vi "Network Steam Read Messages.vi"(8 "error in (no error)":errorcluster, 11 "Model in":refnum<class "Model.lvclass">) -> (0 "error out":errorcluster, 1 "Messages":T1[](array[typedef]), 2 "StillConnected?":bool, 3 "Model out":refnum<class "Model.lvclass">, 4 "Timed Out?":bool)   [LabVIEW 2021, in "Model.lvlib" / "Model.lvclass"]
uses:
  Model.lvclass
  Model.lvclass/Model.ctl
  <userlib>/John_Lib/Network_Streams_Connection/NetworkConnection.lvclass
  4d02eaad-354f-40a9-9b46-312da8ef89df.vi
  <userlib>/John_Lib/Network_Streams_Connection/NetworkCommand--Cluster.ctl
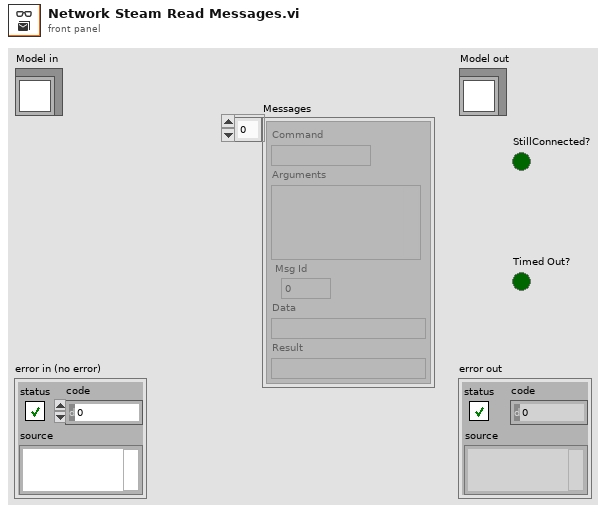
[diagram p1: front panel]
types:
  T1 = typedef "JKI_Network_Streams.lvlib/NetworkConnection.lvclass/NetworkCommand--Cluster.ctl" = cluster{"Command":string, "Arguments":variant, " Msg Id":i32, "Data":string, "Result":string}
  T2 = typedef "Model.lvlib/Model.lvclass/DVR.ctl" = cluster{"JKI_Network_Streams":refnum<class "NetworkConnection.lvclass">}
  T3 = typedef "AMC_FW.lvlib/Queue.ctl" = cluster{"Q":T4, "Name":string}
  T4 = typedef "AMC_FW.lvlib/Message Queue.ctl" = refnum<queue>
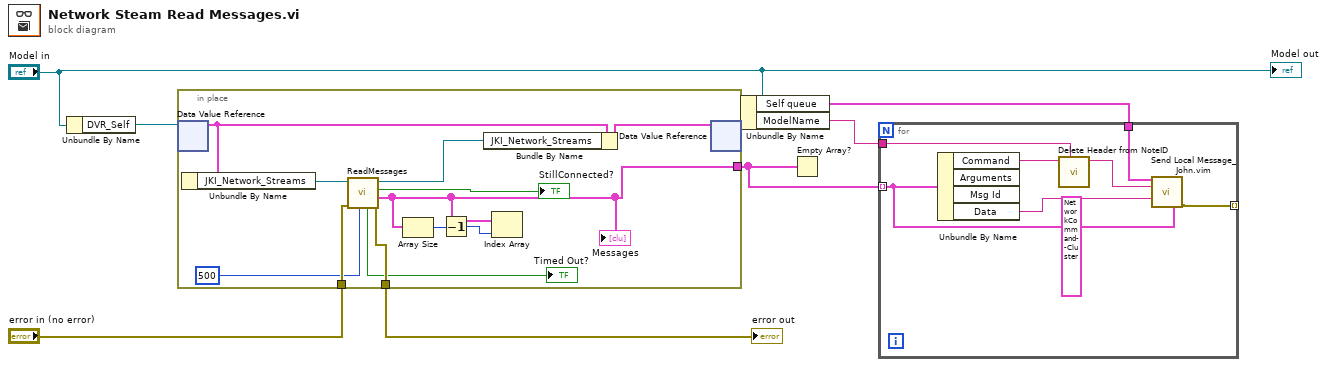
[diagram p0: block diagram]
diagram:
  n1 = Unbundle By Name("Model in") -> ("DVR_Self"=w7:refnum<data-value>)
  n2 = in-place {
    in-place-border: "error in (no error)" -> [w15]
    in-place-border: [w14] -> w5
    in-place-border: [w8] -> w4
    n3 = in-place-dvr #1(w7) -> (w19:T2)  [unwired: 1 out]
    n4 = Unbundle By Name(w19) -> ("JKI_Network_Streams"=w17:refnum<class "NetworkConnection.lvclass">)
    n5 = call <userlib>:"ReadMessages.vi"("Timeout(ms)"=500, "error in (no error)"=w15, "NetworkConnection in"=w17) -> ("error out"=w14:errorcluster, "Messages"=w8:T1[], "StillConnected?"=→"StillConnected?":bool, "NetworkConnection out"=w16:refnum<class "NetworkConnection.lvclass">, "Timed Out?"=→"Timed Out?":bool)  [unwired: 3 in, 1 out]
    "Messages" <- w8
    n6 = Array Size(array=w8) -> (size(s)=w10:i32)
    n7 = Decrement(x=w10) -> (x-1=w9:i32)
    n8 = Bundle By Name(cluster=w19, "JKI_Network_Streams"=w16) -> (w18:T2)
    n9 = Index Array(array=w8, index=w9) -> ()  [unwired: 1 out]
    n10 = in-place-dvr #1(w18) -> ()  [unwired: 2 out]
  }
  "error out" <- w5
  n11 = Unbundle By Name("Model in") -> ("Self queue"=w2:T3, "ModelName"=w1:string)
  n12 = Empty Array?(array=w4) -> ()  [unwired: 1 out]
  n13 = for {
    tunnel: w4 -> [w26] mode=indexing
    tunnel: w2 -> [w25]
    tunnel: w1 -> [w23]
    tunnel: [w21] -> _ mode=indexing
    (unwired) T1 {"Command"="", "Arguments"=variant, " Msg Id"=-1, "Data"="", "Result"=""} ("NetworkCommand")
    n14 = Unbundle By Name(w26) -> ("Command"=w24:string, "Data"=w22:string)  [unwired: 2 out]
    n15 = call <userlib>:"Delete Header from NoteID.vi"("Actor Name"=w23, "node ID full name"=w24) -> ("node ID delete header ns=2;s="=w20:string)  [unwired: 8 in, 1 out]
    n16 = call "Send Local Message_John.vim"("Queue In"=w25, "Elements at Back"=w20, "message value"=w22, "variant"=w26) -> ("error out"=w21:errorcluster)  [unwired: 9 in, 2 out]
  }
  "Model out" <- "Model in"
